vi "N664_Ctrl_Index.vi"(5 "OldVal":variant, 11 "NewVal":variant) -> (4 "Control Ref OUT":refnum<vi>, 8 "N664 Out":T1={"Up N664"=FALSE, "Down N664"=FALSE, "Step Size (um)"=0.001, "Position (mm)"=9.0, "Home"=FALSE, "Save"=FALSE} {"Position (mm)" min=9.0 max=19.0; "Step Size (um)" min=0.001})   [LabVIEW 2014]
uses:
  Type Defs/N664_V2.ctl
panel:
  in  "N664 Data Type":T1={"Up N664"=FALSE, "Down N664"=FALSE, "Step Size (um)"=0.001, "Position (mm)"=9.0, "Home"=FALSE, "Save"=FALSE} {"Position (mm)" min=9.0 max=19.0; "Step Size (um)" min=0.001}
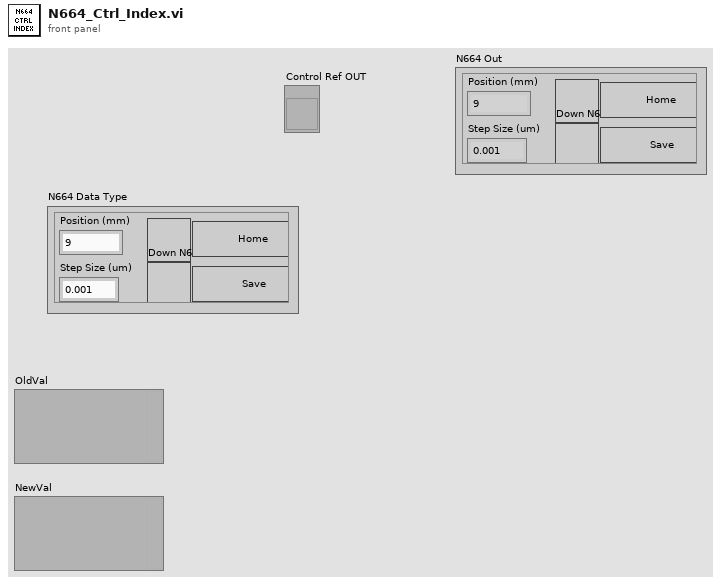
[diagram p1: front panel]
types:
  T1 = typedef "N664_V2.ctl" = cluster{"Up N664":bool, "Down N664":bool, "Step Size (um)":dbl, "Position (mm)":dbl, "Home":bool, "Save":bool}
  T2 = cluster{"Up N664":bool, "Down N664":bool, "Step Size (um)":bool, "Position (mm)":bool, "Home":bool, "Save":bool}
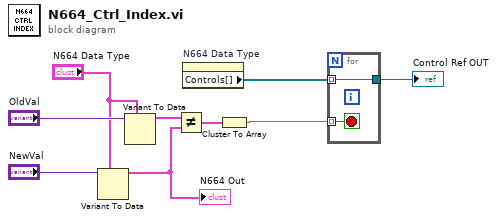
[diagram p0: block diagram]
diagram:
  n1 = Variant To Data(type="N664 Data Type", Variant="NewVal") -> (data=w9:T1)  [unwired: 1 in, 1 out]
  "N664 Out" <- w9
  n2 = Variant To Data(type="N664 Data Type", Variant="OldVal") -> (data=w4:T1)  [unwired: 1 in, 1 out]
  n3 = Not Equal?(x=w4, y=w9) -> (x != y?=w8:T2)
  n4 = property on="N664 Data Type" class="Clust"() -> ("Controls[]"=w1:refnum<vi>[])  [unwired: 2 in, 2 out]
  n5 = Cluster To Array(cluster=w8) -> (array=w5:bool[])
  n6 = for {
    tunnel: w5 -> [w10] mode=indexing
    tunnel: w1 -> [w11] mode=indexing
    tunnel: [w11] -> w3
    stop <- w10 stop-if-true
  }
  "Control Ref OUT" <- w3
